vi "Log Error.vi"(8 "error in":errorcluster, 9 "Source":string, 10 "Code":i32, 11 "Error Log Refnum In":refnum<file>) -> (0 "error out":errorcluster, 3 "Error Log Refnum Out":refnum<file>)   [LabVIEW 2022 SP3]
uses:
  Boiler System Globals.vi
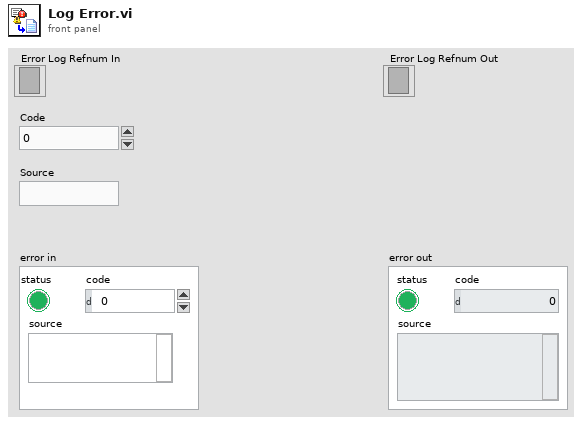
[diagram p1: front panel]
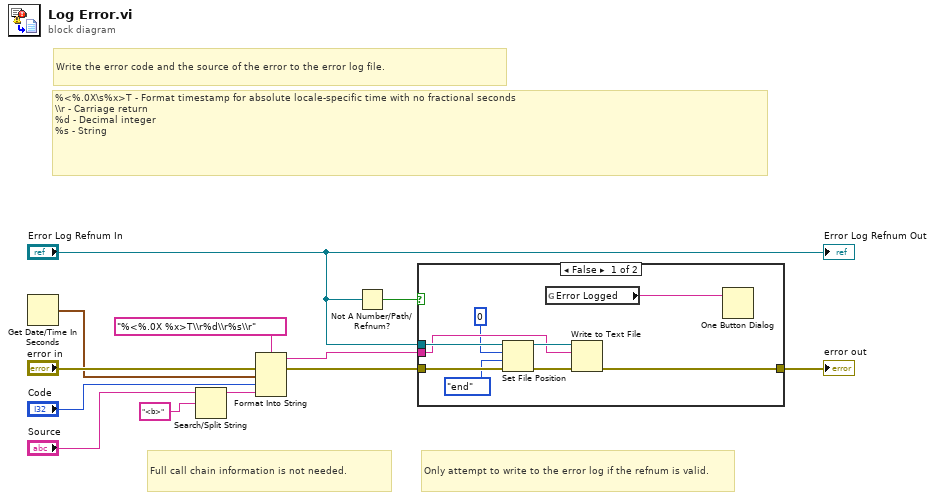
[diagram p0: block diagram]
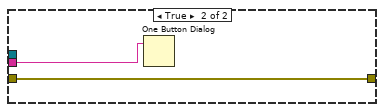
[diagram p2: hidden frame]
diagram:
  # "Full call chain information is not needed."
  # "Only attempt to write to the error log if the refnum is valid."
  # "%<%.0X\\s%x>T - Format timestamp for absolute locale-specific time with no fractional seconds\n\\\\r - Carriage return\n%d - Decimal integer\n%s - String"
  # "Write the error code and the source of the error to the error log file."
  n1 = Get Date/Time In Seconds() -> (seconds since 1Jan1904=w2:timestamp)
  n2 = Search/Split String(string="Source", search string/char (-)="<b>") -> (substring before match=w4:string)  [unwired: 1 in, 2 out]
  n3 = Format Into String(format string="%<%.0X %x>T\\r%d\\r%s\\r", error in="error in", w2, "Code", w4) -> (resulting string=w11:string, error out=w12:errorcluster)  [unwired: 1 in]
  n4 = Not A Number/Path/Refnum?(number/path/refnum="Error Log Refnum In") -> (NaN/Path/Refnum?=w8:bool)
  n5 = case shown="False" w8 {
    tunnel: w12 -> [w17 w23]
    tunnel: w11 -> [w16 w22]
    tunnel: [w21 w23] -> w1
    tunnel: "Error Log Refnum In" -> [w19 _]
    frame False {
      n6 = Set File Position(offset (in bytes) (0)=i64 0, refnum=w19, from (0:start)=enum16{"start", "end", "current"}."end", error in=w17) -> (refnum out=w18:refnum<file>, error out=w20:errorcluster)
      n7 = global read "Boiler System Globals.vi" "Error Logged"() -> (w13:string)
      n8 = Write to Text File(file (use dialog)=w18, text=w16, error in=w20) -> (error out=w21:errorcluster)  [unwired: 1 in, 2 out]
      n9 = One Button Dialog(message=w13) -> ()  [unwired: 1 in, 1 out]
    }
    frame True {
      n10 = One Button Dialog(message=w22) -> ()  [unwired: 1 in, 1 out]
    }
  }
  "error out" <- w1
  "Error Log Refnum Out" <- "Error Log Refnum In"
